vi "GetCRC.vi"(11 "Command":string) -> (3 "CRC":u16 format="%.0x")   [LabVIEW 2012, in "Sierra-M100.lvlib"]
doc: "This VI creates a Circular Redundancy Checksum (CRC) based on the command to send to the mass flow controller. The CRC is 2 bytes long and appeneded to the end of the command and value string along with a carriage return."
uses:
  Sierra-M100.lvlib
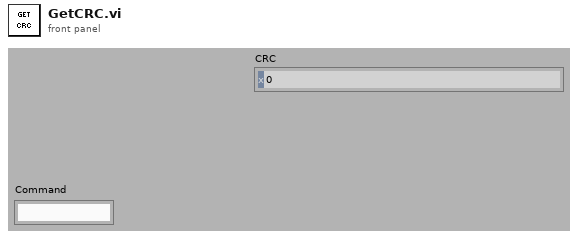
[diagram p1: front panel]
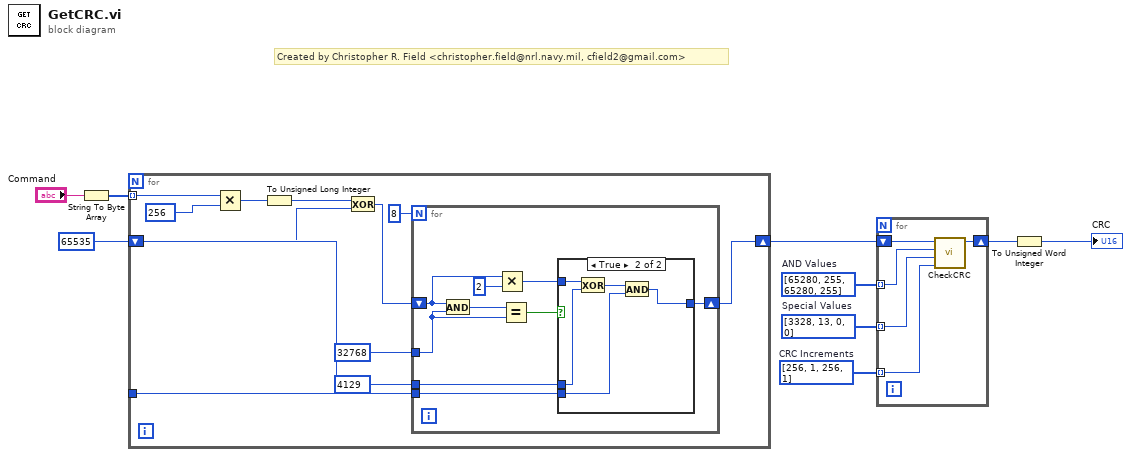
[diagram p0: block diagram]
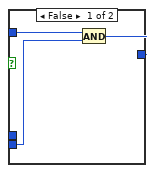
[diagram p2: hidden frame]
diagram:
  w3 = u32[] [256, 1, 256, 1]  # CRC Increments
  w4 = u32[] [3328, 13, 0, 0]  # Special Values
  w5 = u32[] [65280, 255, 65280, 255]  # AND Values
  w7 = u32 65535
  # "Created by Christopher R. Field <christopher.field@nrl.navy.mil, cfield2@gmail.com>"
  n1 = String To Byte Array(string="Command") -> (unsigned byte array=w8:u8[])
  n2 = for {
    shift-right: [w10] -> w6
    shift-left: w7 -> [w16]
    tunnel: w8 -> [w19] mode=indexing
    tunnel: w7 -> [w11]
    n3 = Multiply(x=w19, y=u32 256) -> (x*y=w18:u32)
    n4 = To Unsigned Long Integer(number=w18) -> (unsigned 32bit integer=w17:u32)
    n5 = Exclusive Or(1:w16, 2:w17) -> (0:w14:u32)
    n6 = for {
      N: 8 -> [_]
      tunnel: u32 32768 -> [w28]
      tunnel: u32 4129 -> [w23]
      tunnel: w11 -> [w22]
      shift-right: [w21] -> w10
      shift-left: w14 -> [w26]
      n7 = And(x=w26, y=w28) -> (x .and. y?=w29:u32)
      n8 = Multiply(x=w26, y=u32 2) -> (x*y=w24:u32)
      n9 = Equal?(x=w29, y=w28) -> (x = y?=w25:bool)
      n10 = case shown="True" w25 {
        tunnel: w24 -> [w32 w37]
        tunnel: w23 -> [_ w36]
        tunnel: w22 -> [w31 w34]
        tunnel: [w30 w33] -> w21
        frame False {
          n11 = And(x=w32, y=w31) -> (x .and. y?=w30:u32)
        }
        frame True {
          n12 = Exclusive Or(1:w36, 2:w37) -> (0:w35:u32)
          n13 = And(x=w35, y=w34) -> (x .and. y?=w33:u32)
        }
      }
    }
  }
  n14 = for {
    shift-right: [w41] -> w2
    shift-left: w6 -> [w42]
    tunnel: w5 -> [w40] mode=indexing
    tunnel: w4 -> [w39] mode=indexing
    tunnel: w3 -> [w38] mode=indexing
    n15 = call "CheckCRC.vi"("CRC Increment"=w38, "Special Value"=w39, "AND Value"=w40, "CRC In"=w42) -> ("CRC Out"=w41:u32)  [unwired: 7 in]
  }
  n16 = To Unsigned Word Integer(number=w2) -> (unsigned 16bit integer=→"CRC":u16)
